vi "NumberOfRegistersToRead.vi"(8 "Error In":errorcluster, 11 "Measurement TextRing":u16) -> (0 "Error Out":errorcluster, 3 "Numer of Registers":u16)   [LabVIEW 2018, in "SensorPlugins.lvlib" / "SiemensDigitalEnergyMeter.lvclass"]
uses:
  SiemensDigitalEnergyMeter.lvclass
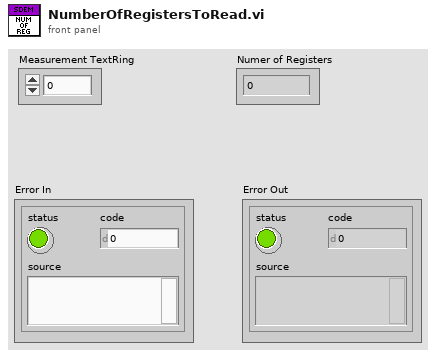
[diagram p1: front panel]
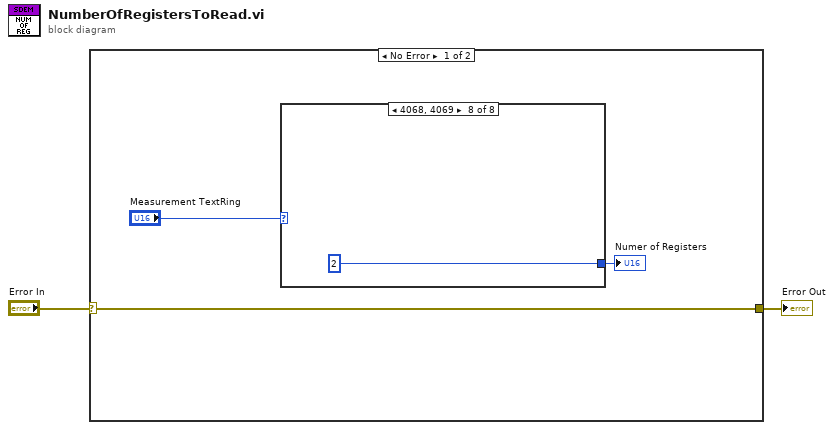
[diagram p0: block diagram]
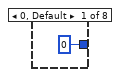
[diagram p2: hidden frame]
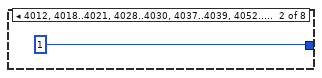
[diagram p3: hidden frame]
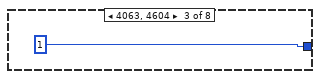
[diagram p4: hidden frame]
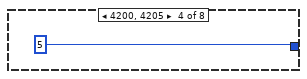
[diagram p5: hidden frame]
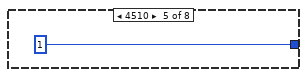
[diagram p6: hidden frame]
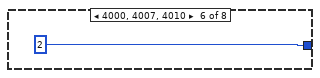
[diagram p7: hidden frame]
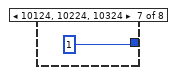
[diagram p8: hidden frame]
diagram:
  n1 = case shown="No Error" "Error In" {
    selector: "Error In" -> [w3 w14]
    tunnel: [w3 w14] -> w1
    frame No Error {
      n2 = case shown="4068, 4069" "Measurement TextRing" {
        tunnel: [u16 0 ("x") u16 1 ("x") u16 1 ("x") u16 5 ("x") u16 1 ("x") u16 2 ("x") u16 1 ("y") u16 2 ("x")] -> w4
        frame 0, Default {
        }
        frame 4012, 4018..4021, 4028..4030, 4037..4039, 4052..4060 {
        }
        frame 4063, 4604 {
        }
        frame 4200, 4205 {
        }
        frame 4510 {
        }
        frame 4000, 4007, 4010 {
        }
        frame 10124, 10224, 10324 {
        }
        frame 4068, 4069 {
        }
      }
      "Numer of Registers" <- w4
    }
    frame Error {
    }
  }
  "Error Out" <- w1
